vi "Configure Record Data.vi"(8 "error in (no error)":errorcluster, 9 "Data Composition (0: Composite Sample Waveform)":u16(ring) items=["Composite Sample Waveform", "Composite Peak Detect Waveform", "Singular Sample Waveform"], 10 "Data Resolution (0: Full)":u16(ring) items=["Full Waveform", "Reduced Waveform"], 11 "VISA resource name":refnum<visa-resource-name>) -> (0 "error out":errorcluster, 3 "VISA resource name out":refnum<visa-resource-name>)   [LabVIEW 2009, in "Tektronix DPO MSO 2000 4000 Series.lvlib"]
doc: "Configures the data settings for the DPO2K and MSO2K series instruments.\n\n<B>Note:</B>\n\nThis VI is not valid for DPO 3k, MSO 3k, DPO 4k and MSO 4k Series."
uses:
  <instrlib>/Tektronix DPO MSO 2000 4000 Series/Tektronix DPO MSO 2000 4000 Series.lvlib
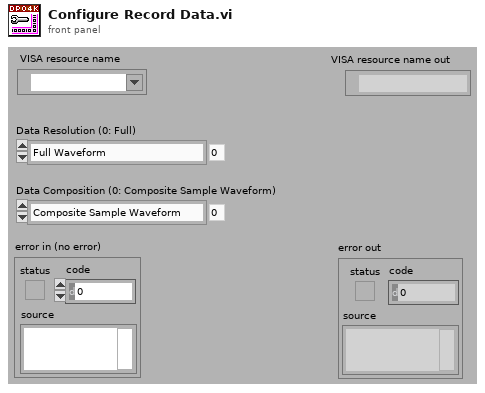
[diagram p1: front panel]
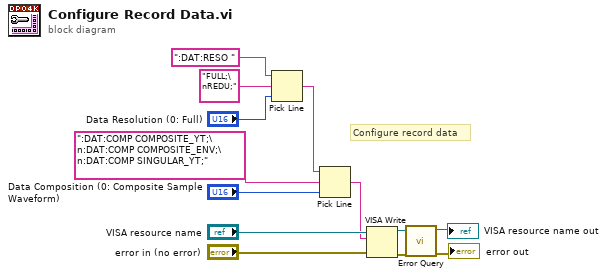
[diagram p0: block diagram]
diagram:
  # "Configure record data"
  n1 = Pick Line(string ("")=":DAT:RESO ", multi-line string="FULL;\nREDU;" ("Data Resolution Options"), line index="Data Resolution (0: Full)") -> (output string=w3:string)
  n2 = Pick Line(string ("")=w3, multi-line string=":DAT:COMP COMPOSITE_YT;\n:DAT:COMP COMPOSITE_ENV;\n:DAT:COMP SINGULAR_YT;", line index="Data Composition (0: Composite Sample Waveform)") -> (output string=w1:string)
  n3 = VISA Write(VISA resource name="VISA resource name", write buffer=w1, error in (no error)="error in (no error)") -> (VISA resource name out=w9:refnum<visa-resource-name>, error out=w8:errorcluster)  [unwired: 1 out]
  n4 = call <instrlib>:"Error Query.vi"("error in (no error)"=w8, "VISA resource name"=w9) -> ("error out"=→"error out":errorcluster, "VISA resource name out"=→"VISA resource name out":refnum<visa-resource-name>)  [unwired: 6 in, 2 out]
